vi "Read Tree Ref Top Left Visible Cell No Error.vi"(11 "TreeRef":refnum<vi>) -> (2 "TopLeft":T1, 3 "TreeRef":refnum<vi>)   [LabVIEW 2020, in "BetterDragAndDrop.lvlib" / "BetterTreeHandle.lvclass"]
uses:
  Classes/BetterTreeHandle/BetterTreeHandle.lvclass
  <vilib>/Utility/miscctls.llb/LVNodeAndColumnTypeDef.ctl
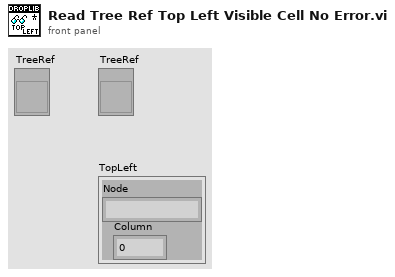
[diagram p1: front panel]
types:
  T1 = typedef "LVNodeAndColumnTypeDef.ctl" = cluster{"Node":string, "Column":i32}
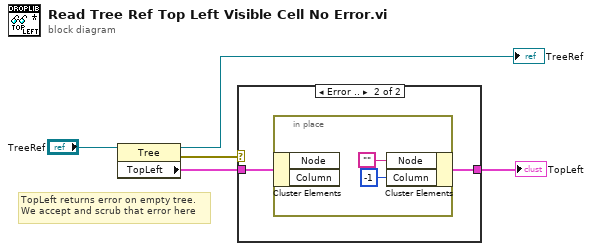
[diagram p0: block diagram]
diagram:
  # "TopLeft returns error on empty tree.\nWe accept and scrub that error here"
  n1 = property class="Tree"(reference="TreeRef") -> (reference out=→"TreeRef":refnum<vi>, error out=w4:errorcluster, "TopLeft"=w3:T1)  [unwired: 1 in]
  n2 = case shown="Error .." w4 {
    tunnel: w3 -> [w6 w8]
    tunnel: [w6 w7] -> w2
    frame No Error {
    }
    frame Error {
      n3 = in-place {
        n4 = in-place-cluster #1(w8) -> ()  [unwired: 2 out]
        n5 = in-place-cluster #1("Node"="", "Column"=-1) -> (w7:T1)
      }
    }
  }
  "TopLeft" <- w2
